vi "OFDM_ControlledChannel_Estimation.vi"() -> ()   [LabVIEW 2015]
uses:
  <vilib>/imath/engines/lvmath/Plug In/_Char/NIMS_CH_character datatype.ctl
  <vilib>/Analysis/2dsp.llb/Inverse Complex FFT.vi
  <vilib>/Analysis/2dsp.llb/Complex FFT.vi
  <vilib>/addons/Modulation/Digital/General/MT Generate Bits (Fibonacci, PN Order).vi
  <vilib>/addons/Modulation/Digital/General/MT Generate QAM System Parameters(M).vi
  <vilib>/addons/Modulation/Digital/General/MT Map Bits to QAM Symbols.vi
  <vilib>/imath/engines/lvmath2/RunTimeEngine/RangeToken/NIMS_Range.vi
  <instcachedir>/0/NIMS_Range_D919CC09935940E88F755EC1C6F49AC1.lvgen/NIMS_Range_D919CC09935940E88F755EC1C6F49AC1_001.vi
  <vilib>/imath/engines/lvmath2/RunTimeEngine/BuiltInFunctions/sets_diff/NIMS_sets_diff(GV2).vi
  <instcachedir>/0/NIMS_sets_diff(GV2)_CE188B9DAFCC49368CD9C62F83DF72AA.lvgen/NIMS_sets_diff(GV2)_CE188B9DAFCC49368CD9C62F83DF72AA_007.vi
  <vilib>/imathl/engines/lvmath/Functions/Error Handling/Create Error.vi
  <vilib>/imath/engines/lvmath2/RunTimeEngine/BuiltInFunctions/rand/NIMS_rand(1,I32).vi
  <vilib>/imath/engines/lvmath2/RunTimeEngine/ErrorHandling/NIMS_Error From Error Code.vi
  <vilib>/imath/engines/lvmath2/RunTimeEngine/IndexReplace/NIMS V(V)=V.vi
  <instcachedir>/0/NIMS V(V)=V_422D7BAD0B0F4E4DA085EB3347135799.lvgen/NIMS V(V)=V_422D7BAD0B0F4E4DA085EB3347135799_000.vi
  <vilib>/imath/engines/lvmath2/RunTimeEngine/IndexRead/NIMS V(R2).vi
  <instcachedir>/0/NIMS V(R2)_C76619605A0E4E9F8B2FA9389712AC47.lvgen/NIMS V(R2)_C76619605A0E4E9F8B2FA9389712AC47_002.vi
  <instcachedir>/0/NIMS V(R2)_C76619605A0E4E9F8B2FA9389712AC47.lvgen/NIMS V(R2)_C76619605A0E4E9F8B2FA9389712AC47_001.vi
  <instcachedir>/0/NIMS V(V)=V_422D7BAD0B0F4E4DA085EB3347135799.lvgen/NIMS V(V)=V_422D7BAD0B0F4E4DA085EB3347135799_001.vi
  <vilib>/imath/engines/lvmath2/RunTimeEngine/ErrorHandling/NIMS_Create Error From Enums.vi
  <vilib>/imath/engines/lvmath2/RunTimeEngine/NodeEndStatement/NIMS_NodeEndStatement_Output.vi
  <instcachedir>/0/NIMS_NodeEndStatement_Output_53EC0D466D134D7ABD903AC30B43404B.lvgen/NIMS_NodeEndStatement_Output_53EC0D466D134D7ABD903AC30B43404B_010.vi
  <instcachedir>/0/NIMS_NodeEndStatement_Output_53EC0D466D134D7ABD903AC30B43404B.lvgen/NIMS_NodeEndStatement_Output_53EC0D466D134D7ABD903AC30B43404B_000.vi
  <vilib>/imath/engines/lvmath2/RunTimeEngine/ErrorHandling/NIMS_Finalize Error.vi
  <vilib>/imath/engines/lvmath2/RunTimeEngine/Managers/WorkSpace/UID Generator.vi
  <vilib>/imath/engines/lvmath2/RunTimeEngine/BuiltInFunctions/figure/NIMS_figure.vi
  <vilib>/imath/engines/lvmath/Plug In/_Char/NIMS_CH_Character RV to String.vi
  <vilib>/imath/engines/lvmath2/RunTimeEngine/IndexRead/NIMS V(S).vi
  <instcachedir>/0/NIMS V(S)_0488751826AF41519A22953C041130DC.lvgen/NIMS V(S)_0488751826AF41519A22953C041130DC_002.vi
  <vilib>/imath/engines/lvmath2/RunTimeEngine/BuiltInFunctions/abs/NIMS_abs(signed).vi
  <instcachedir>/0/NIMS_abs(signed)_C4FCB8E6058B49B797C7C8D53CA5F6EC.lvgen/NIMS_abs(signed)_C4FCB8E6058B49B797C7C8D53CA5F6EC_006.vi
  <vilib>/imath/engines/lvmath2/RunTimeEngine/BuiltInFunctions/plot/NIMS_plot(G, Str).vi
  <instcachedir>/0/NIMS_plot(G, Str)_4C4ED324FCF14F2FB79D7E74DE209E0D.lvgen/NIMS_plot(G, Str)_4C4ED324FCF14F2FB79D7E74DE209E0D_000.vi
  <vilib>/imath/engines/lvmath2/RunTimeEngine/BuiltInFunctions/hold/NIMS_hold(Enums).vi
  <vilib>/imath/engines/lvmath2/RunTimeEngine/BuiltInFunctions/legend/NIMS_legend(Arb).vi
  <vilib>/imath/engines/lvmath2/RunTimeEngine/BuiltInFunctions/title/NIMS_title.vi
  <vilib>/imath/engines/lvmath2/RunTimeEngine/BuiltInFunctions/xlabel/NIMS_xlabel.vi
  <vilib>/imath/engines/lvmath2/RunTimeEngine/BuiltInFunctions/ylabel/NIMS_ylabel.vi
  <vilib>/addons/Modulation/niDMT.lvlib
  <vilib>/Analysis/NI_AALPro.lvlib
panel:
  in  "multipath":i32=4
  out "BER":dbl
  out "H_est":cdb[](array[numeric])=[0.3124502508916735-1.0659025548913155i, 0.3098883648124847-0.9973440941865369i, 0.2944585577793801-0.9302408777414778i, 0.2691602140526042-0.8640548774968628i, 0.2409595441959415-0.7977497473136677i, 0.21682275877317667-0.730289141052868i, 0.2022505745619648-0.6609401273192841i, 0.1968817331954435-0.590183433693114i, 0.19888948252062089-0.5188032024983996i, 0.20644707038450516-0.44758357605918375i, 0.21809500975433796-0.3772250810962436i, 0.2338428740782951-0.30809378191729697i, 0.25406750192478583-0.2404721272267966i, 0.27914573186221947-0.17464256572919531i, 0.30933249892644754-0.11090023304388594i, 0.34439512402309047-0.04959101245002163i, 0.3839790245252108+0.00892652585830448i, 0.4277296178058714+0.0642938116869992i, 0.4753054965386392+0.11617188474095969i, 0.5264179545990988+0.16430022432104438i, 0.5807914611633394+0.20843791962710206i, 0.63815048540745+0.2483440598589815i, 0.6982022117278903+0.2837937023995898i, 0.7605846854026027+0.31462577736406727i, 0.8249186669299001+0.3406951830506126i, 0.8908249168080955+0.3618568177574244i, 0.9579220223446281+0.37798561533335606i, 1.0258198780834407+0.3890366518298797i, 1.094126205377603+0.39498503884912206i, 1.162448725580184+0.3958058879932099i, 1.2303964851034601+0.3914941565518747i, 1.2975838305965346+0.3821241845652664i, 1.363626433767718+0.3677901577611399i, 1.4281399663253205+0.34858626186724956i, 1.4907479624813367+0.3246252093330858i, 1.551105406462499+0.29609381949508135i, 1.6088751449992225+0.2631974384114043i, 1.663720024821924+0.22614141214022299i, 1.7153157419916163+0.18514644849048448i, 1.7633893898917004+0.1404947022742514i, 1.807680911236174+0.09248369005436526i, 1.8479302487390354+0.04141092839366753i, 1.8838942612269924-0.012415213047552907i, 1.915397471977594-0.06864295221921751i, 1.9422813203810982-0.12690965397380038i, 1.9643872458277645-0.18685268316377562i, 1.9815760991095266-0.2481040662821022i, 1.9937863766250192-0.3102744763836789i, 2.000975986174552-0.3729692481638892i, 2.003102835558436-0.4357937163181169i, 2.0001450188584338-0.4983538953818152i, 1.992161375282127-0.5602585192507157i, 1.9792309303185487-0.6211170016606194i, 1.9614327094567339-0.6805387563473276i, 1.9388648828353199-0.738139870872094i, 1.911702199191357-0.793563128097982i, 1.8801385519114981-0.8464579847135076i, 1.8443678343823968-0.896473897407187i, 1.8046003158993236-0.943272433917915i, 1.7611117693920189-0.9865636061861037i, 1.7141943436988405-1.026069537202544i, 1.6641401876581465-1.0615123499580261i, 1.6112535643795507-1.092630674900684i, 1.5558871940576906-1.1192291723080183i, 1.4984059111584602-1.141129009914873i, 1.4391745501477529-1.1581513554560916i, 1.3785646731155417-1.1701368446036775i, 1.316974752648112-1.1770039847782734i, 1.2548099889558288-1.1786907513376819i, 1.1924755822490571-1.1751351196397055i, 1.1303774161990578-1.1662957865314778i, 1.0689241083206782-1.1522143348174565i, 1.008524959589662-1.1329530687914302i, 0.9495892709817526-1.108574292747187i, 0.8925208526121632-1.0791604560325434i, 0.8377015511539831-1.0448745882114228i, 0.7855077224197715-1.0058998639017769i, 0.7363157222220873-0.9624194577215566i, 0.6904906524251236-0.9146343190254478i, 0.6483525990996136-0.8628164961150737i, 0.6102103943679245-0.8072558120287919i, 0.5763728703524237-0.7482420898049603i, 0.5471327618664675-0.6860789557042896i, 0.522718414487368-0.621125248876903i, 0.5033420764834258-0.5537536116952773i, 0.48921599612294164-0.484336686531889i, 0.4805328320720499-0.4132556793973201i, 0.4774068845882189-0.34092605085457456i, 0.4799328643267506-0.26777182510476183i, 0.4882054819429469-0.19421702634899132i, 0.5022980337757369-0.1206881800104046i, 0.5221981588985588-0.04762181640027122i, 0.5478720820684779+0.02454303294810707i, 0.5792860280425596+0.09536733650142859i, 0.6163848239579237+0.1644159274992249i, 0.6590277064719077+0.23126909827236053i, 0.707052514621904+0.29551100592453333i, 0.7602970874453046+0.3567258075594411i, 0.8185797400186542+0.4145076459493834i, 0.8816406915751089+0.46849060654106656i, 0.949200637386977+0.5183187604497989i, 1.0209802727265676+0.5636361787908883i, 1.0966843548168093+0.604102263291344i, 1.1759538886831145+0.6394377381249777i, 1.258413941301515+0.6693786580773026i, 1.3436895796480435+0.693661077933831i, 1.4313949376707964+0.7120404848924526i, 1.5211004172061262+0.7243500958005615i, 1.6123654870624486+0.7304425599179287i, 1.7047496160481808+0.730170526504325i, 1.7978073471492246+0.723408572841839i, 1.8910735200614295+0.7101189883018317i, 1.9840780486581289+0.6902859902779819i, 2.076350846812659+0.663893796163968i, 2.167423406622568+0.6309492135088207i, 2.256833533082266+0.5915494104829757i, 2.344120609410378+0.5458141454122208i, 2.428824018825527+0.49386317662234347i, 2.5104911729594743+0.43583760975372954i, 2.588701597096529+0.37196393970515773i, 2.663042844934137+0.3024900086900053i, 2.7331024701697415+0.22766365892164933i, 2.7984819022523726+0.14775102309763338i, 2.8588380736373904+0.06309139585216708i, 2.9138417925317386-0.025957637696373582i, 2.963163867142361-0.11903849242961258i, 3.006493725655977-0.21577991734041993i, 3.043595276178414-0.3157559978666502i, 3.0742510467952737-0.41852715355740394i, 3.09824356559216-0.523653803961782i, 3.1153772131753827-0.6306885142068297i, 3.125543780234084-0.7391524317313731i, 3.1286569099781136-0.8485588495521832i, 3.1246302456173214-0.9584210606860305i, 3.1134007220212716-1.0682510186582623i, 3.0949984406983875-1.1775553190285306i, 3.069476794816805-1.285839217865063i, 3.0368891775446625-1.392607971236088i, 2.9973117889746517-1.4973721691864046i, 2.9509120568976828-1.5996637376670968i, 2.8978802160292227-1.6990199366058205i, 2.8384065010847377-1.7949780259302306i, 2.7727015773412154-1.887086871431893i, 2.701057832321732-1.974941762358012i, 2.6237880841108847-2.0581495938197034i, 2.5412051507932722-2.1363172609280823i, 2.453638205565061-2.2090686073483226i, 2.3614818420686934-2.276095270961834i, 2.26514700905818-2.337105838204084i, 2.1650446552875313-2.391808895510542i, 2.061596646787244-2.4399339412251995i, 1.9552685186937573-2.481294121326142i, 1.8465367234199939-2.515723493699979i, 1.735877713378878-2.5430561162333203i, 1.6237725104504626-2.5631492084654113i, 1.5107204143833157-2.5759526365460483i, 1.3972252943931358-2.5814394282776627i, 1.2837910196956206-2.5795826114626874i, 1.1709193008963479-2.5703787218522574i, 1.05910321416042-2.553918326992318i, 0.9488336770428196-2.5303155023775195i, 0.8406016070985292-2.4996843235025095i, 0.7348892171146753-2.4621607873067495i, 0.6321439008069609-2.4179685765089505i, 0.532804347123233-2.367353295272637i, 0.43730924501133855-2.310560547761332i, 0.3460827606737934-2.247854474534134i, 0.25949096933179006-2.179573361732439i, 0.1778854234611898-2.10607403189322i, 0.10161767553785406-2.027713307553447i, 0.0310201518071848-1.9448616482045533i, -0.03365122640725378-1.8579440611558196i, -0.09215966401235694-1.7673991906709876i, -0.14426836591501996-1.6736656810137989i, -0.18976267606257818-1.5771898178163608i, -0.22851649456412731-1.478448452184237i, -0.260425860569203-1.3779260765913555i, -0.2853868132273412-1.276107183511645i, -0.30331868544049767-1.1734773002592718i, -0.31423398512030853-1.0705260935093504i, -0.31816851393083023-0.9677442647772334i, -0.31515807353611885-0.8656225155782732i, -0.3052610438517941-0.764645993046406i, -0.2886261177997286-0.6652776267899027i, -0.2654245665533585-0.5679747920356177i, -0.2358276612861198-0.4731948640104057i, -0.20002644686017146-0.3813833711100433i, -0.15829106289256428-0.2929384544059954i, -0.11091142268907189-0.2082464081386491i, -0.058177439555468-0.1276935265483914i, -0.0003952267408924917-0.051649804147990315i, 0.062064302732049874+0.01957996346026219i, 0.12881403589738816+0.08570728040169319i, 0.19946685978915135+0.14644365080162983i, 0.2736275044163836+0.2015229220523187i, 0.3508680716881894+0.25076831461368476i, 0.4307525064886881+0.2940253922125724i, 0.5128447537019994+0.33113971857582614i, 0.5966974622288814+0.36197216135263865i, 0.6818180970366469+0.38644480388159536i, 0.767702827109247+0.4044950334236299i, 0.8538478214306333+0.416060237239676i, 0.9397797421767795+0.4211264886237226i, 1.0251472242917496+0.41987460500198037i, 1.1096293959116301+0.41253408983371537i, 1.1929053851725064+0.3993344465781937i, 1.2745595642736265+0.3804274486067811i, 1.3537972816668784+0.355653948939243i, 1.4297291298673123+0.32477707050744425i, 1.501465701389978+0.28755993624325i, 1.5685190126955444+0.24414917876416337i, 1.6320067760271613+0.19622546943024002i, 1.6934481275735975+0.14585298928717375i, 1.7543622035236224+0.09509591938065831i, 1.8160110147464825+0.045667745537330884i, 1.8786280708333114-0.0021208272923766563i, 1.9421897560556998-0.0483097893770756i, 2.0066724546852965-0.09293913098541838i, 2.072052550993693-0.13604884238601578i, 2.1383064292525-0.17767891384749285i, 2.205410473733308-0.21786933563846253i, 2.273341068707767-0.2566600980275737i, 2.3420745984474682-0.2940911912834392i, 2.411587447224022-0.33020260567468374i, 2.4818559993090172-0.365034331469922i, 2.5528566389741076-0.39862635893779963i, 2.6245657504908824-0.43101867834693103i, 2.696959718130951-0.46225127996594095i, 2.7700149261659033-0.4923641540634456i, 2.843707758867393-0.5213972909080876i, 2.918014600507009-0.549390680768483i, 2.992911835356362-0.5763843139132563i, 3.0683758476870393-0.602418180611025i, 3.1443830217706967-0.6275322711304295i, 3.220909741878923-0.6517665757400867i, 3.297932392283328-0.6751610847086215i, 3.3754273572555227-0.6977557883046587i, 3.453371021067093-0.7195906767968169i, 3.531739767989698-0.7407057404537339i, 3.6105099822949236-0.7611409695440281i, 3.689658048254381-0.7809363543363242i, 3.7691603501396567-0.8001318850992416i, 3.8489932722224083-0.8187675521014165i, 3.9291331987742235-0.8368833456114679i, 4.009556514066712-0.8545192558980209i, 4.090239602371461-0.8717152732296952i, 4.171158847960128-0.888511387875126i, 4.2522906351043-0.9049475901029327i, 4.333611348075589-0.9210638701817405i, 4.415097371145579-0.9369002183801695i, 4.496725088585931-0.9524966249668538i, 4.57847088466823-0.967893080210414i, 4.660311143664087-0.9831295743794747i, 4.742222249845087-0.9982460977426562i, 4.824180587482892-1.0132826405685922i, 4.906162540849085-1.0282791931259037i]
  out "OFDM_output_recv":cdb[][](array[numeric])
  out "Demod Bits":i8[](array[numeric])
  out "OFDM Frame":cdb[](array[numeric])
  in  "cp_length":i16=28
  in  "frame_length":i64=220
  in  "pilot_offset_time":i16=4
  in  "pilot_offset_freq":i16=12
  in  "pilot_start":i16=2
  in  "SC_pilot":i16=18
  in  "SC_data":i64=180
  in  "SC_total":i16=256
  out "Bit Stream":i8[](array[numeric])
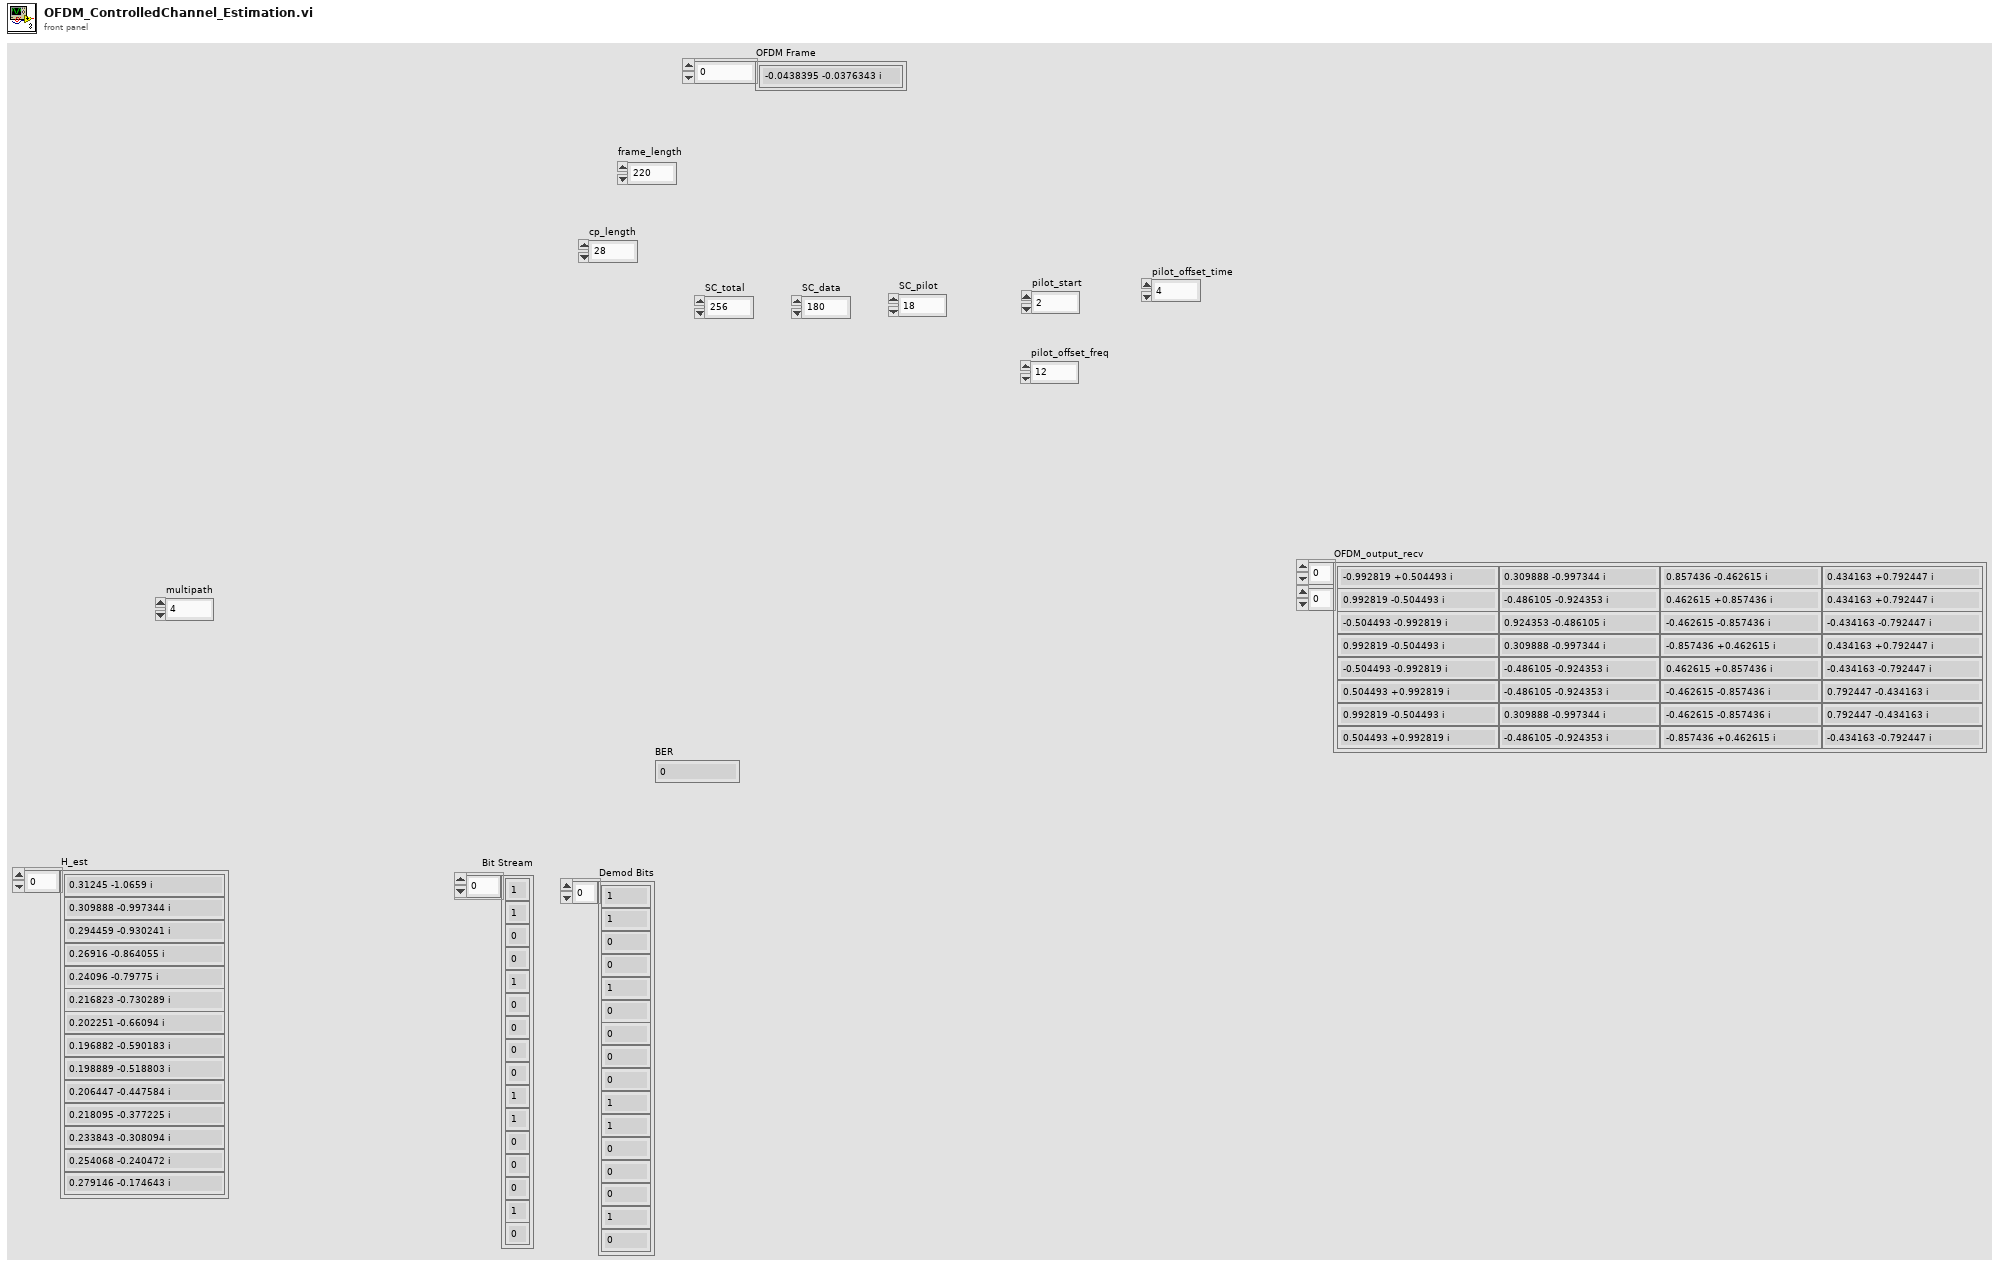
[diagram p1: front panel]
types:
  T1 = cluster{"samples per symbol (16)":i32, "symbol map":cdb[]}
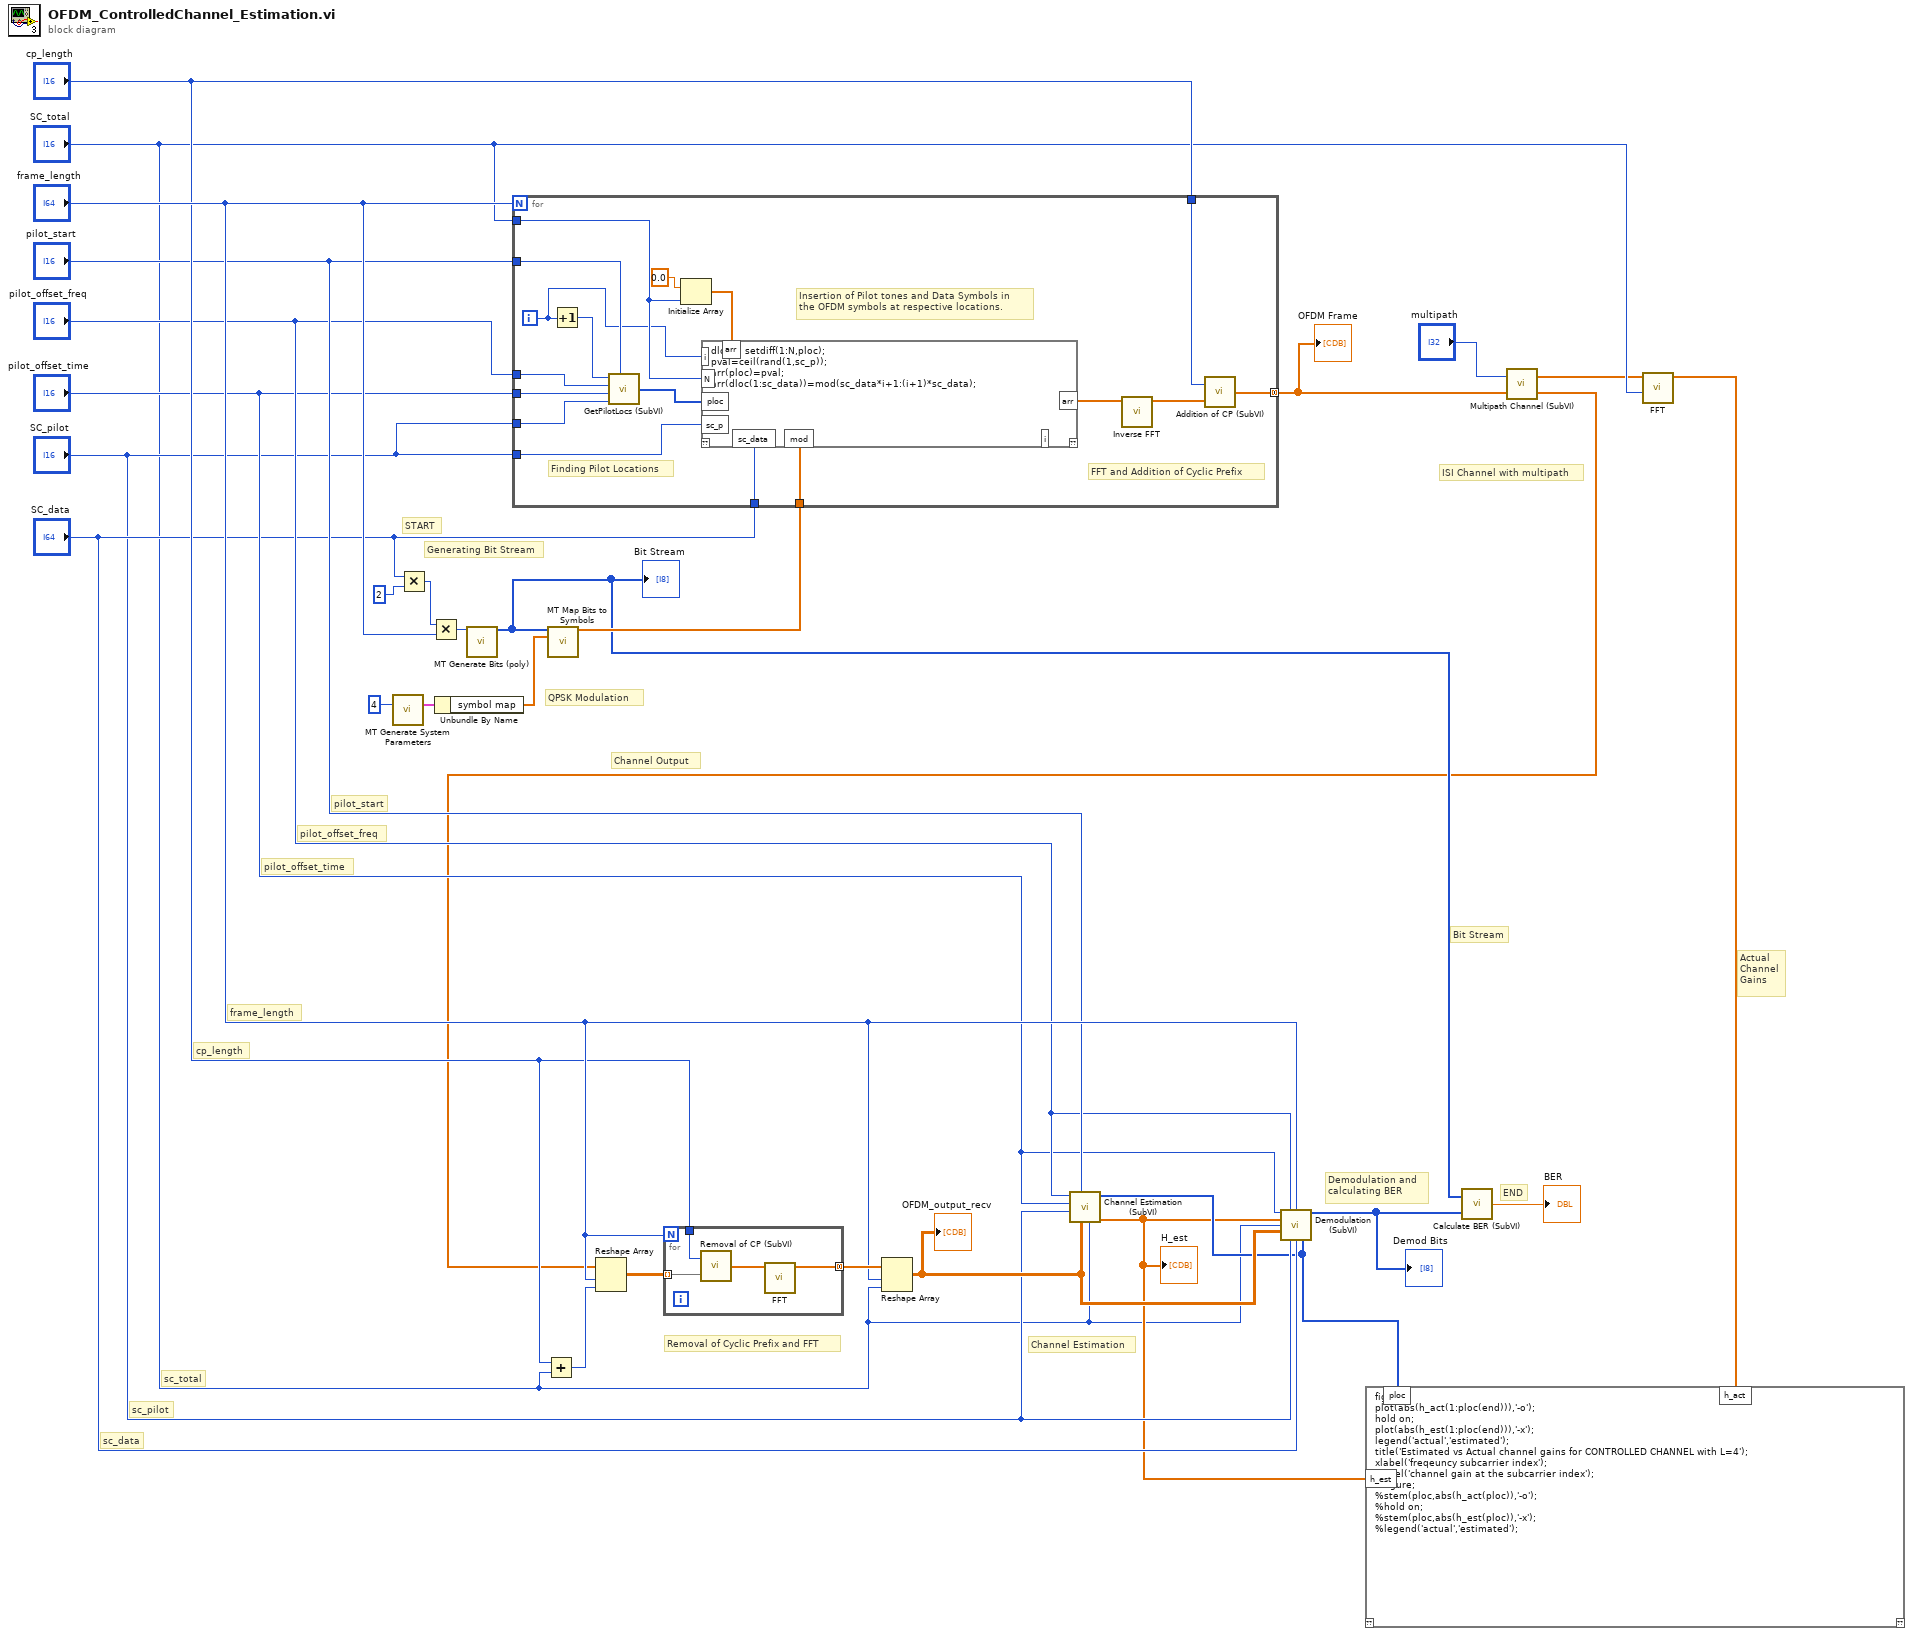
[diagram p0: block diagram]
diagram:
  # "Actual\nChannel\nGains"
  # "ISI Channel with multipath"
  # "Bit Stream"
  # "Channel Output"
  # "START"
  # "Generating Bit Stream"
  # "QPSK Modulation"
  # "pilot_offset_time"
  # "pilot_offset_freq"
  # "pilot_start"
  # "END"
  # "Demodulation and\ncalculating BER"
  # "Channel Estimation"
  # "Removal of Cyclic Prefix and FFT"
  # "cp_length"
  # "frame_length"
  # "sc_total"
  # "sc_pilot"
  # "sc_data"
  n1 = call-poly <vilib>:"MT Generate System Parameters.vi"("M-QAM (16)"=4) -> ("QAM system parameters"=w24:T1)  [unwired: 12 in, 2 out]
  n2 = Multiply(x="SC_data", y=i64 2) -> (x*y=w27:i64)
  n3 = Multiply(x=w27, y="frame_length") -> (x*y=w28:i64)
  n4 = Unbundle By Name(w24) -> ("symbol map"=w23:cdb[])
  n5 = call-poly <vilib>:"MT Generate Bits (poly).vi"("total bits (128)"=w28) -> ("output bit stream"=w11:i8[])  [unwired: 12 in, 2 out]
  "Bit Stream" <- w11
  n6 = Add(x="cp_length", y="SC_total") -> (x+y=w21:i16)
  n7 = call-poly <vilib>:"MT Map Bits to Symbols.vi"("input bit stream"=w11, "symbol map"=w23) -> ("symbols"=w26:cdb[])  [unwired: 12 in, 1 out]
  n8 = for {
    N: "frame_length" -> [_]
    tunnel: "pilot_offset_time" -> [w46]
    tunnel: "pilot_offset_freq" -> [w45]
    tunnel: "pilot_start" -> [w44]
    tunnel: "SC_pilot" -> [w38]
    tunnel: "SC_pilot" -> [w37]
    tunnel: "SC_total" -> [w35]
    tunnel: "SC_data" -> [w33]
    tunnel: w26 -> [w32]
    tunnel: "cp_length" -> [w31]
    tunnel: [w30] -> w3 mode=concatenating
    i -> [w34]
    # "FFT and Addition of Cyclic Prefix"
    # "Insertion of Pilot tones and Data Symbols in \nthe OFDM symbols at respective locations."
    # "Finding Pilot Locations"
    n9 = Increment(x=w34) -> (x+1=w36:i32)
    n10 = call "GetPilotLocs (SubVI).vi"("sym #"=w36, "pilot_offset_freq"=w45, "pilot_offset_time"=w46, "sc_pilot"=w38, "pilot_start"=w44) -> ("Array"=w43:i32[])
    n11 = Initialize Array(0.0 ("element"), w35) -> (w41:dbl[])
    n12 = mathscript code="dloc = setdiff(1:N,ploc);\npval=ceil(rand(1,sc_p));\narr(ploc)=pval;\narr(dloc(1:sc_data))=mod(sc_data*i+1:(i+1)*sc_data);"("ploc"=w43, "N"=w35, "arr"=w41, "sc_p"=w37, "mod"=w32, "sc_data"=w33, "i"=w34) -> ("arr"=w40:cdb[])  [unwired: 1 in, 2 out]
    n13 = call-poly <vilib>:"Inverse FFT.vi"("FFT {X}"=w40) -> ("X"=w39:cdb[])  [unwired: 9 in, 1 out]
    n14 = call "Addition of CP (SubVI).vi"("ifft_output"=w39, "cp_length"=w31) -> ("ifft_output with CP"=w30:cdb[])
  }
  "OFDM Frame" <- w3
  n15 = call "Multipath Channel (SubVI).vi"("OFDM Frame"=w3, "multipath"="multipath") -> ("ch_op"=w2:cdb[], "tap_gain_vec"=w1:cdb[])
  n16 = Reshape Array(w2, "frame_length", w21) -> (w13:cdb[][])
  n17 = for {
    N: "frame_length" -> [_]
    tunnel: w13 -> [w186] mode=indexing
    tunnel: "cp_length" -> [w185]
    tunnel: [w183] -> w22 mode=concatenating
    n18 = call "Removal of CP (SubVI).vi"("ch_output in"=w186, "cp_length"=w185) -> ("ch_output out"=w184:cdb[])
    n19 = call-poly <vilib>:"FFT.vi"("X"=w184) -> ("FFT {X}"=w183:cdb[])  [unwired: 9 in, 1 out]
  }
  n20 = Reshape Array(w22, "frame_length", "SC_total") -> (w20:cdb[][])
  "OFDM_output_recv" <- w20
  n21 = call "Channel Estimation (SubVI).vi"("SC_total"="SC_total", "ofdm_output"=w20, "pilot_start"="pilot_start", "SC_pilot"="SC_pilot", "pilot_offset_time"="pilot_offset_time", "pilot_offset_freq"="pilot_offset_freq") -> ("H_est"=w7:cdb[], "est_ploc_mtx"=w8:i32[])  [unwired: 1 in, 3 out]
  "H_est" <- w7
  n22 = call "Demodulation (SubVI).vi"("pilot_offset_time"="pilot_offset_time", "pilot_offset_freq"="pilot_offset_freq", "frame_length"="frame_length", "H_est"=w7, "SC_total"="SC_total", "OFDM_output"=w20, "SC_pilot"="SC_pilot", "SC_data"="SC_data", "est_ploc_mtx"=w8) -> ("demod_data"=w12:i8[])  [unwired: 6 in]
  "Demod Bits" <- w12
  n23 = call "Calculate BER (SubVI).vi"("Original Bits"=w12, "Demod Bits"=w11) -> ("BER"=→"BER":dbl)
  n24 = call-poly <vilib>:"FFT.vi"("FFT size"="SC_total", "X"=w1) -> ("FFT {X}"=w6:cdb[])  [unwired: 8 in, 1 out]
  n25 = mathscript code="figure;\nplot(abs(h_act(1:ploc(end))),'-o');\nhold on;\nplot(abs(h_est(1:ploc(end))),'-x');\nlegend('actual','estimated');\ntitle('Estimated vs Actual channel gains for CONTROLLED CHANNEL with L=4');\nxlabel('freqeuncy subcarrier index');\nylabel('channel gain at the subcarrier index');\n%figure;\n%stem(ploc,abs(h_act(ploc)),'-o');\n%hold on;\n%stem(ploc,abs(h_est(ploc)),'-x');\n%legend('actual','estimated');"("h_est"=w7, "ploc"=w8, "h_act"=w6) -> ()  [unwired: 1 in, 1 out]
